vi "StringToAutoData.vi"(11 "String":string) -> (2 "Path File Names":string[](array[string]), 3 "Auto":T1)   [LabVIEW 2018]
uses:
  AutoFileDataType.ctl
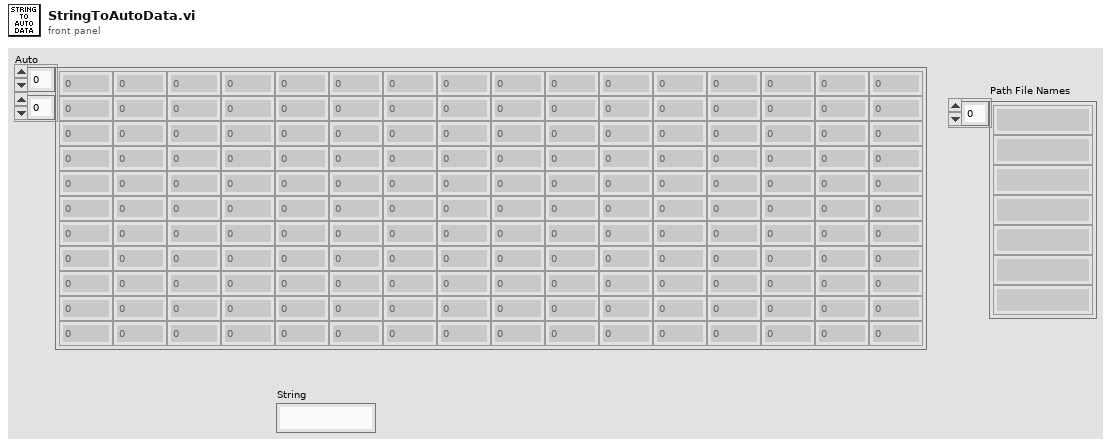
[diagram p1: front panel]
types:
  T1 = typedef "AutoFileDataType.ctl" = dbl[][]
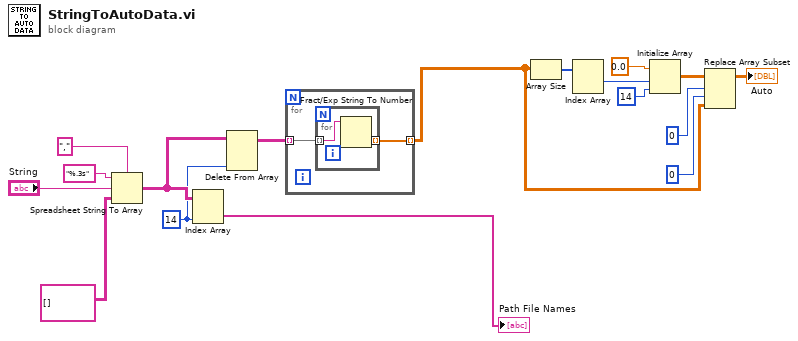
[diagram p0: block diagram]
diagram:
  w3 = 14 ("disabled index (col)")
  n1 = Spreadsheet String To Array(delimiter (Tab)=",", format string="%.3s", spreadsheet string="String", array type (2D Dbl)=string[][] [] ("Path File Names 2")) -> (array=w4:string[][])
  n2 = Index Array(array=w4, index (col)=w3) -> (element=→"Path File Names":string[])  [unwired: 1 in]
  n3 = Delete From Array(array=w4, index (col)=w3) -> (array with subset deleted=w2:string[][])  [unwired: 2 in, 1 out]
  n4 = for {
    tunnel: w2 -> [w19] mode=indexing
    tunnel: [w18] -> w1 mode=indexing
    n5 = for {
      tunnel: w19 -> [w21] mode=indexing
      tunnel: [w20] -> w18 mode=indexing
      n6 = Fract/Exp String To Number(string=w21) -> (number=w20:dbl)  [unwired: 3 in, 1 out]
    }
  }
  n7 = Array Size(array=w1) -> (size(s)=w13:i32[])
  n8 = Index Array(array=w13) -> (element #1=w8:i32)  [unwired: 2 in, 1 out]
  n9 = Initialize Array(0.0 ("element"), w8, 14 ("dimension size")) -> (w12:dbl[][])
  n10 = Replace Array Subset(array=w12, new element=w1, index (row)=0, index (col)=0 ("disabled index (col)")) -> (→"Auto":dbl[][])
